vi "BBR_2022.vi"() -> ()   [LabVIEW 2021]
panel:
  out "Total Lift":dbl format="%#_4g"
  out "RPM":dbl format="%#_2g"
  in  "stop":bool
  out "voltage":dynamicdata(graph)
  out "Red and Green":dynamicdata(graph)
  out "Blue and Pink":dynamicdata(graph)
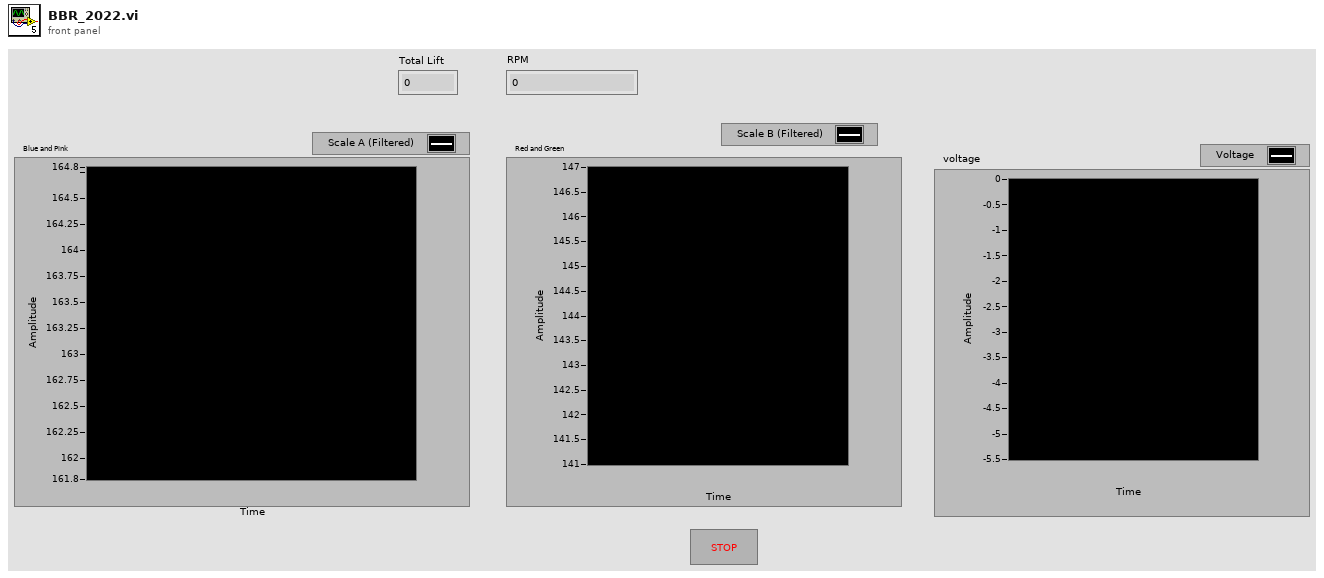
[diagram p1: front panel]
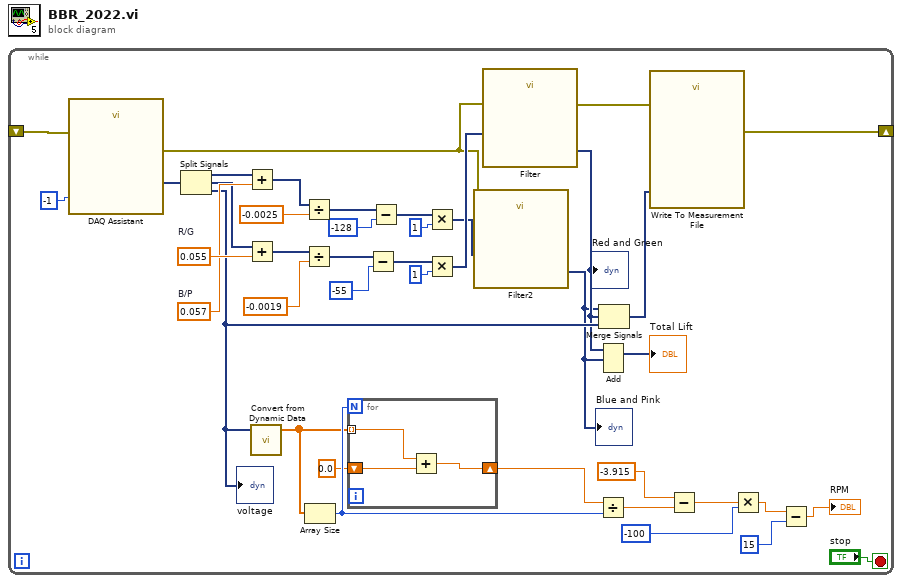
[diagram p0: block diagram]
diagram:
  n1 = while {
    shift-right: [w5] -> _
    shift-left: _ -> [w19]
    stop <- "stop" stop-if-true
    w38 = 0.057  # B/P
    w39 = 0.055  # R/G
    n2 = call "DAQ Assistant"("timeout (s)"=-1, "error in"=w19) -> ("data"=w35:dynamicdata, "error out"=w6:errorcluster)  [unwired: 14 in, 2 out]
    n3 = Split Signals(w35) -> (w33:dynamicdata, w34:dynamicdata, w21:dynamicdata)  [unwired: 3 in]
    "voltage" <- w21
    n4 = Add(x=w33, y=w38) -> (x+y=w41:dynamicdata)
    n5 = Add(x=w34, y=w39) -> (x+y=w40:dynamicdata)
    n6 = call "Convert from Dynamic Data"("Dynamic Data Type"=w21) -> ("Array"=w15:dbl[])  [unwired: 3 in]
    n7 = Divide(x=w41, y=-0.0025) -> (x/y=w32:dynamicdata)
    n8 = Divide(x=w40, y=-0.0019) -> (x/y=w30:dynamicdata)
    n9 = Array Size(array=w15) -> (size(s)=w18:i32)
    n10 = for {
      N: w18 -> [_]
      shift-right: [w42] -> w17
      shift-left: 0.0 -> [w44]
      tunnel: w15 -> [w43] mode=indexing
      n11 = Add(x=w43, y=w44) -> (x+y=w42:dbl)
    }
    n12 = Subtract(x=w30, y=-55) -> (x-y=w25:dynamicdata)
    n13 = Subtract(x=w32, y=-128) -> (x-y=w26:dynamicdata)
    n14 = Multiply(x=w26, y=1) -> (x*y=w8:dynamicdata)
    n15 = Multiply(x=w25, y=1) -> (x*y=w24:dynamicdata)
    n16 = call "Filter2"("error in (no error)"=w6, "Signal"=w8) -> ("Filtered Signal"=w7:dynamicdata)  [unwired: 8 in, 1 out]
    "Blue and Pink" <- w7
    n17 = call "Filter"("error in (no error)"=w6, "Signal"=w24) -> ("error out"=w4:errorcluster, "Filtered Signal"=w10:dynamicdata)  [unwired: 8 in]
    "Red and Green" <- w10
    n18 = Add(1:w7, 2:w10) -> (0:→"Total Lift":dynamicdata)  [unwired: 1 in, 1 out]
    n19 = Divide(x=w17, y=w18) -> (x/y=w12:dbl)
    n20 = Merge Signals(w7, w10, w21) -> (w22:dynamicdata)
    n21 = call "Write To Measurement File"("Signals"=w22, "error in (no error)"=w4) -> ("error out"=w5:errorcluster)  [unwired: 15 in, 2 out]
    n22 = Subtract(x=-3.915, y=w12) -> (x-y=w13:dbl)
    n23 = Multiply(x=w13, y=-100) -> (x*y=w3:dbl)
    n24 = Subtract(x=w3, y=15) -> (x-y=→"RPM":dbl)
  }
